vi "Enumerer tilkoblede comporter.vi"(11 "error in (no error)":errorcluster) -> (8 "Com port w Select string":string[](array[string]), 10 "Valid interface found":bool, 14 "Port names":string[](array[string]), 15 "error out":errorcluster)   [LabVIEW 2011]
panel:
  # "Allow debug must be on to get the correct lists... Go figure"
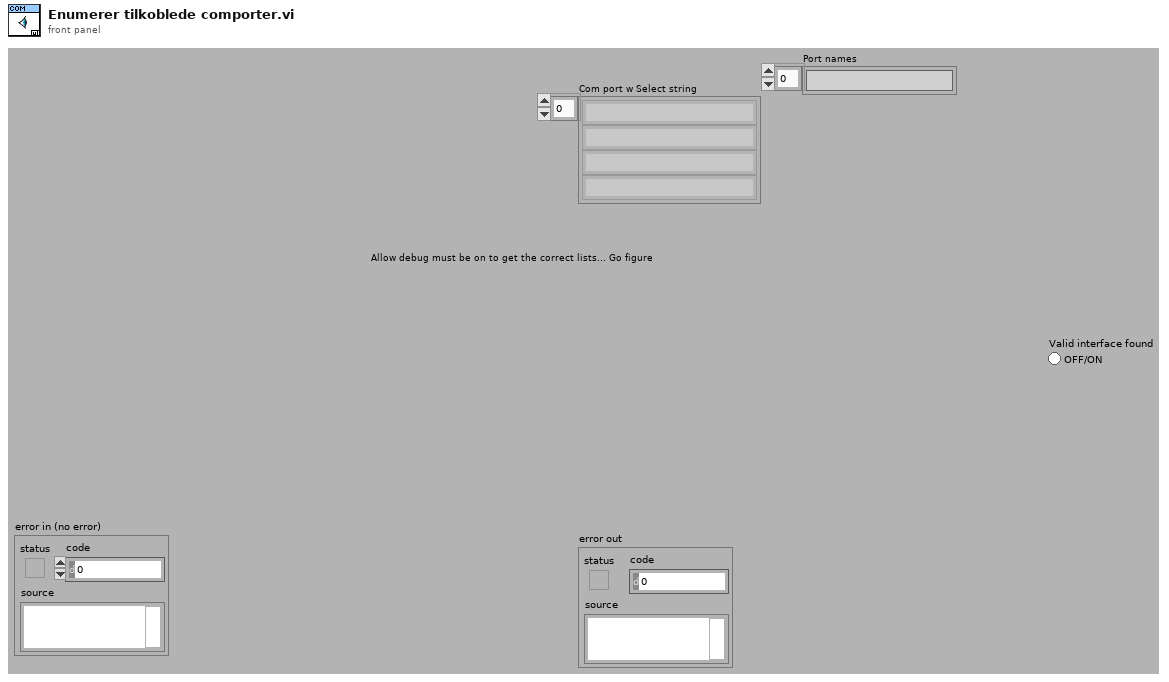
[diagram p1: front panel]
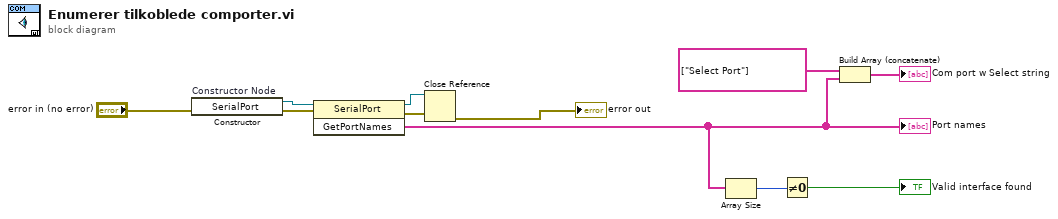
[diagram p0: block diagram]
diagram:
  n1 = constructor on="Constructor Node" class="SerialPort"(error in="error in (no error)") -> (reference out=w3:refnum<k24>, error out=w6:errorcluster)  [unwired: 2 in, 1 out]
  n2 = invoke class="SerialPort" method="GetPortNames"(reference=w3, error in=w6) -> (reference out=w4:refnum<k24>, error out=w5:errorcluster, "GetPortNames"=w7:string[])  [unwired: 1 in]
  "Port names" <- w7
  n3 = Close Reference(reference=w4, error in (no error)=w5) -> (error out=→"error out":errorcluster)
  n4 = Array Size(array=w7) -> (size(s)=w1:i32)
  n5 = Not Equal To 0?(x=w1) -> (x != 0?=→"Valid interface found":bool)
  n6 = Build Array (concatenate)(string[] ["Select Port"], w7) -> (→"Com port w Select string":string[])
